vi "בדיקת מתח שחרור של סליל פיקוד ללא עומס 4.vi"(7 "resultUserPrompt":bool=TRUE, 8 "error":errorcluster, 11 "Path for Log":path) -> (0 "error out":errorcluster, 1 "מצב ממסר פתוח/סגור":bool, 2 "מתח פתיחת הממסר":dbl format="%.4f", 3 "מתח מוצא מהספק":dbl format="%.4f")   [LabVIEW 2014]
uses:
  <vilib>/DAQmx/create/channels.llb/DAQmx Create Channel (DO-Digital Output).vi
  <vilib>/DAQmx/write.llb/DAQmx Write (Digital Bool 1Line 1Point).vi
panel:
  out "progress":dbl(slide) scale=0.0..11.0
  out "error IO DMM":errorcluster
  in  "Stop Button":bool
  # "Right-Click to\nexplain error"
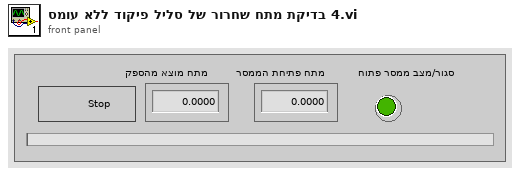
[diagram p1: front panel]
types:
  T1 = enum32{"Invalid", "Standard", "Closed", "Hidden", "Minimized", "Maximized"}
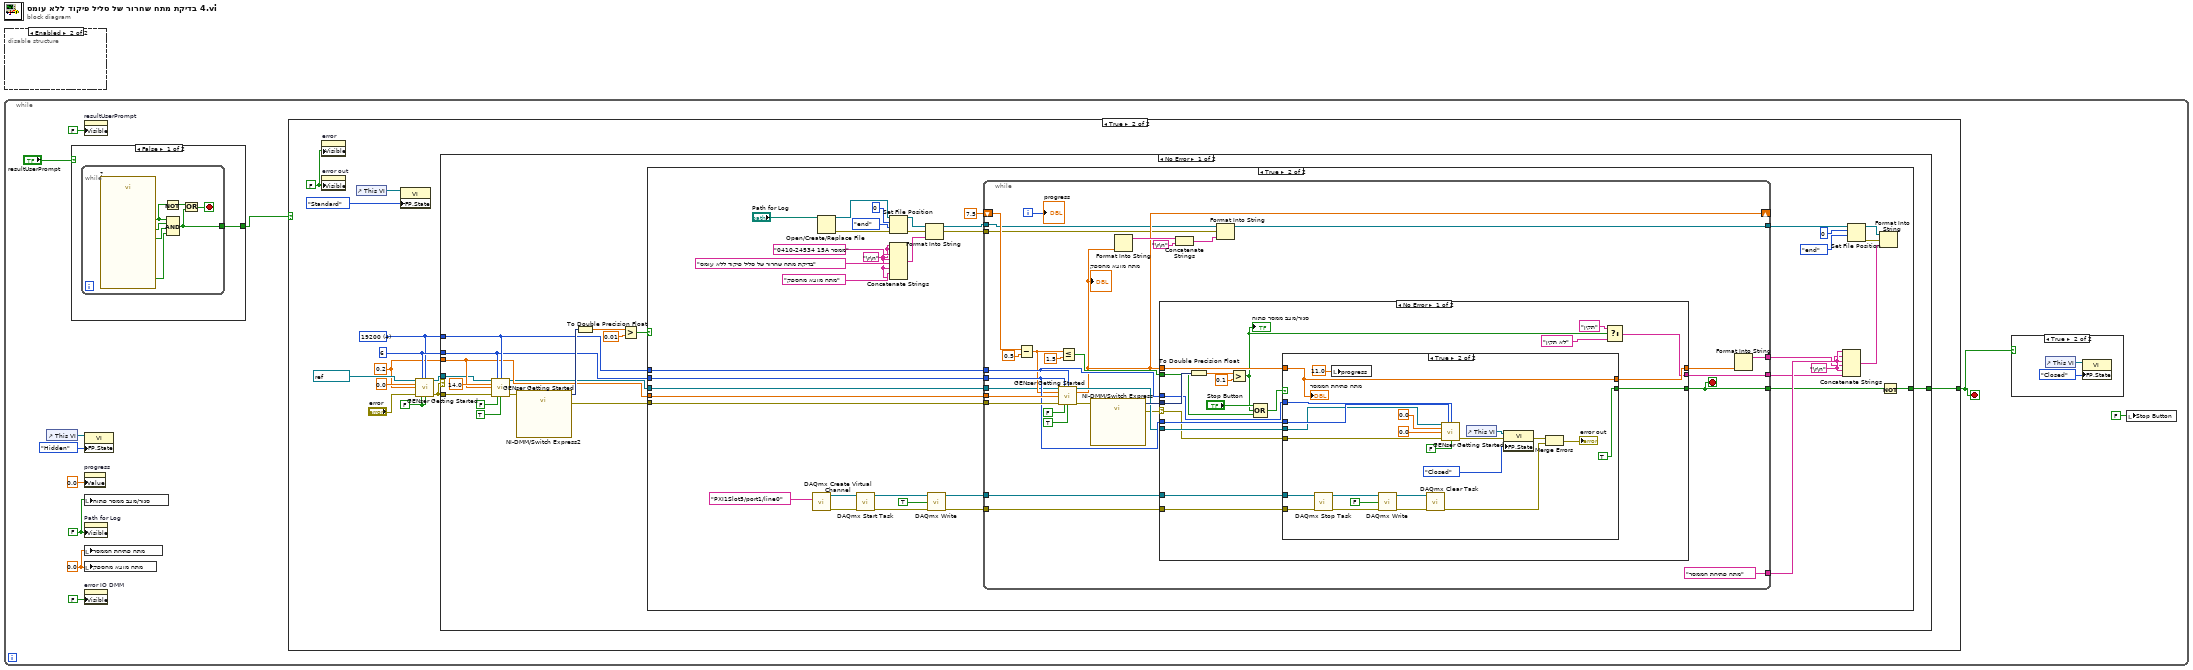
[diagram p0: block diagram]
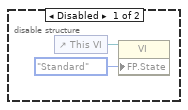
[diagram p2: hidden frame]
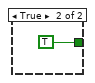
[diagram p4: hidden frame]
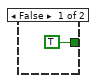
[diagram p5: hidden frame]
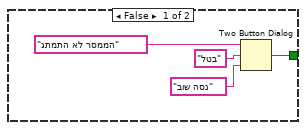
[diagram p6: hidden frame]
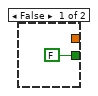
[diagram p7: hidden frame]
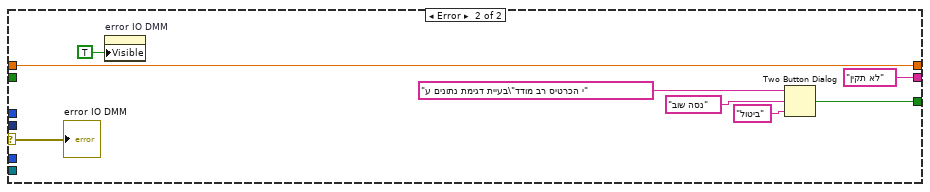
[diagram p8: hidden frame]
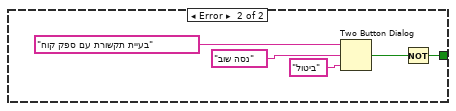
[diagram p9: hidden frame]
diagram:
  n1 = disable-structure shown="Enabled" {
    frame Disabled {
      n2 = control-ref of="This VI"() -> (w1:refnum<vi>)
      n3 = property class="VI"(reference=w1, "FP.State"=T1."Standard" ("Front Panel Window:State")) -> ()  [unwired: 1 in, 2 out]
    }
    frame Enabled {
    }
  }
  n4 = while {
    stop <- w3 stop-if-true
    w7 = FALSE ("מגע סגור")
    w10 = 0.0 ("signals out")
    n5 = control-ref of="This VI"() -> (w9:refnum<vi>)
    n6 = case shown="False" "resultUserPrompt" {
      tunnel: [w16 TRUE] -> w4
      frame False {
        n7 = while {
          tunnel: [w17] -> w16
          stop <- w20 stop-if-true
          n8 = call "?"() -> ("הדקי הרב מודד"=w21:bool, "(מגע שלילי (מעטפת"=w22:bool, "A מגע חיובי"=w23:bool, "OK"=w18:bool)  [unwired: 15 in, 1 out]
          n9 = Not(x=w18) -> (.not. x?=w19:bool)
          n10 = Compound Arithmetic op=AND(w18, w23, w22, w21) -> (w17:bool)
          n11 = Or(x=w19, y=w17) -> (x .or. y?=w20:bool)
        }
      }
      frame True {
      }
    }
    n12 = property on="resultUserPrompt" class="Bool (strict)"("Visible"=FALSE) -> ()  [unwired: 2 in, 2 out]
    n13 = property class="VI"(reference=w9, "FP.State"=T1."Hidden" ("Front Panel Window:State")) -> ()  [unwired: 1 in, 2 out]
    n14 = property on="progress" class="Slide (strict)"("Value"=0.0 ("progress")) -> ()  [unwired: 2 in, 2 out]
    n15 = local write "מצב ממסר פתוח/סגור"(w7) -> ()
    n16 = property on="Path for Log" class="Path"("Visible"=w7) -> ()  [unwired: 2 in, 2 out]
    n17 = local write "מתח פתיחת הממסר"(w10) -> ()
    n18 = local write "מתח מוצא מהספק"(w10) -> ()
    n19 = property on="error IO DMM" class="Clust (strict)"("Visible"=FALSE) -> ()  [unwired: 2 in, 2 out]
    n20 = case shown="True" w4 {
      tunnel: [TRUE ("T button?") w30] -> w3
      frame False {
      }
      frame True {
        w28 = FALSE ("Visible")
        w29 = FALSE ("Output On (T)")
        w34 = u16 4 items=["1200", "2400", "4800", "9600", "19200"] ("BAUD")
        w35 = i16 6 ("GEN Addr")
        w31 = 0.2 ("Current Limit")
        n21 = property on="error" class="Clust (strict)"("Visible"=w28) -> ()  [unwired: 2 in, 2 out]
        n22 = property on="error out" class="Clust (strict)"("Visible"=w28) -> ()  [unwired: 2 in, 2 out]
        n23 = control-ref of="This VI"() -> (w26:refnum<vi>)
        n24 = property class="VI"(reference=w26, "FP.State"=T1."Standard" ("Front Panel Window:State")) -> ()  [unwired: 1 in, 2 out]
        n25 = call "GENser Getting Started.vi"("VISA"=refnum<visa-resource-name> "COM6", "GEN Addr"=w35, "BAUD"=w34, "Voltage Limit"=0.0, "Current Limit"=w31, "error"="error", "Reset (T)"=w29, "Output On (T)"=w29) -> ("VISA out"=w36:refnum<visa-resource-name>, "error out"=w37:errorcluster)  [unwired: 4 in, 2 out]
        n26 = case shown="No Error" w37 {
          tunnel: w37 -> [w47 _]
          tunnel: w36 -> [w43 _]
          tunnel: w35 -> [w45 _]
          tunnel: w34 -> [w46 _]
          tunnel: w31 -> [w44 _]
          tunnel: [w39 w182] -> w30
          frame No Error {
            n27 = call "GENser Getting Started.vi"("VISA"=w43, "GEN Addr"=w45, "BAUD"=w46, "Voltage Limit"=14.0, "Current Limit"=w44, "error"=w47, "Reset (T)"=FALSE, "Output On (T)"=TRUE) -> ("VISA out"=w42:refnum<visa-resource-name>, "error out"=w51:errorcluster)  [unwired: 4 in, 2 out]
            n28 = call "NI-DMM/Switch Express2"("error in"=w51) -> ("signals out"=w50:dynamicdata, "error out"=w48:errorcluster)  [unwired: 16 in, 1 out]
            n29 = To Double Precision Float(number=w50) -> (double precision float=w41:dbl)
            n30 = Greater?(x=w41, y=0.01) -> (0:w49:bool)
            n31 = case shown="True" w49 {
              tunnel: w48 -> [_ w98]
              tunnel: w45 -> [_ w97]
              tunnel: w46 -> [_ w96]
              tunnel: w44 -> [_ w95]
              tunnel: w42 -> [_ w93]
              tunnel: [w55 w59] -> w39
              frame False {
                n32 = Two Button Dialog(message="הממסר לא התמתג", 1:"נסה שוב" ("T button name (\"OK\")"), 2:"בטל" ("T button name (\"OK\")")) -> (T button?=w55:bool)
              }
              frame True {
                w69 = "\r\n"
                w92 = "\r\n"
                n33 = call-poly <vilib>:"DAQmx Create Virtual Channel.vi"("lines"=tag "PXI1Slot5/port1/line0") -> ("task out"=w67:refnum<k21>, "error out"=w68:errorcluster)  [unwired: 13 in]
                n34 = Open/Create/Replace File(file path (use dialog)="Path for Log") -> (refnum out=w80:refnum<file>, error out=w79:errorcluster)  [unwired: 5 in, 1 out]
                n35 = call <vilib>:"DAQmx Start Task.vi"("task/channels in"=w67, "error in"=w68) -> ("task out"=w65:refnum<k21>, "error out"=w64:errorcluster)  [unwired: 12 in]
                n36 = Set File Position(offset (in bytes) (0)=i64 0, refnum=w80, from (0:start)=enum16{"start", "end", "current"}."end", error in=w79) -> (refnum out=w75:refnum<file>, error out=w70:errorcluster)
                n37 = Concatenate Strings(w69, w69, "0410-24534 15A ממסר", w69, "בדיקת מתח שחרור של סליל פיקוד ללא עומס", w69, "מתח מוצא מהספק", w69) -> (w78:string)
                n38 = Format Into String(initial string=w75, error in=w70, w78) -> (resulting string=w72:refnum<file>, error out=w71:errorcluster)  [unwired: 1 in]
                n39 = call-poly <vilib>:"DAQmx Write.vi"("task/channels in"=w65, "data"=TRUE, "error in"=w64) -> ("task out"=w62:refnum<k21>, "error out"=w61:errorcluster)  [unwired: 10 in, 1 out]
                n40 = while {
                  tunnel: w98 -> [w129]
                  tunnel: w97 -> [w122]
                  tunnel: w96 -> [w121]
                  tunnel: w95 -> [w127]
                  shift-right: [w104] -> _
                  shift-left: 7.5 ("y") -> [w125]
                  tunnel: w93 -> [w114]
                  tunnel: [w109] -> w87
                  tunnel: ["מתח פתיחת הממסר"] -> w86
                  tunnel: [w107] -> w85
                  tunnel: [w106] -> w84
                  tunnel: w72 -> [w103]
                  tunnel: w71 -> [w102]
                  tunnel: w62 -> [w101]
                  tunnel: w61 -> [w100]
                  tunnel: [w99] -> w60
                  i -> [w115]
                  stop <- w99 stop-if-true
                  n41 = Subtract(x=w125, y=0.5) -> (x-y=w118:dbl)
                  n42 = call "GENser Getting Started.vi"("VISA"=w114, "GEN Addr"=w122, "BAUD"=w121, "Voltage Limit"=w118, "Current Limit"=w127, "error"=w129, "Reset (T)"=FALSE, "Output On (T)"=TRUE) -> ("VISA out"=w120:refnum<visa-resource-name>, "Output Voltage"=w104:dbl, "error out"=w124:errorcluster)  [unwired: 4 in, 1 out]
                  "מתח מוצא מהספק" <- w104
                  n43 = Less Or Equal?(x=w118, y=1.5) -> (x <= y?=w117:bool)
                  n44 = call "NI-DMM/Switch Express"("error in"=w124) -> ("signals out"=w123:dynamicdata, "error out"=w116:errorcluster)  [unwired: 16 in, 1 out]
                  n45 = Format Into String(w104) -> (resulting string=w111:string)  [unwired: 3 in, 1 out]
                  n46 = case shown="No Error" w116 {
                    selector: w116 -> [w139 w180]
                    tunnel: w123 -> [w148 _]
                    tunnel: [w145 w176] -> w99
                    tunnel: w122 -> [w144 _]
                    tunnel: w121 -> [w143 _]
                    tunnel: w120 -> [w142 _]
                    tunnel: w117 -> [w141 _]
                    tunnel: w104 -> [w140 w174]
                    tunnel: [w133 w174] -> w110
                    tunnel: [w132 "לא תקין"] -> w106
                    tunnel: w101 -> [w131 _]
                    tunnel: w100 -> [w130 _]
                    frame No Error {
                      n47 = To Double Precision Float(number=w148) -> (double precision float=w138:dbl)
                      n48 = Greater?(x=w138, y=0.1) -> (0:w134:bool)
                      "מצב ממסר פתוח/סגור" <- w134
                      n49 = Compound Arithmetic op=OR("Stop Button", w134, w141) -> (w147:bool)
                      n50 = case shown="True" w147 {
                        tunnel: [FALSE TRUE] -> w145
                        tunnel: w144 -> [_ w171]
                        tunnel: w143 -> [_ w170]
                        tunnel: w142 -> [_ w169]
                        tunnel: w139 -> [_ w166]
                        tunnel: w140 -> [_ w160]
                        tunnel: [_ w160] -> w133
                        tunnel: w131 -> [_ w154]
                        tunnel: w130 -> [_ w153]
                        frame False {
                        }
                        frame True {
                          n51 = call <vilib>:"DAQmx Stop Task.vi"("task/channels in"=w154, "error in"=w153) -> ("task out"=w159:refnum<k21>, "error out"=w158:errorcluster)  [unwired: 12 in]
                          n52 = local write "progress"(11.0 ("progress")) -> ()
                          n53 = call-poly <vilib>:"DAQmx Write.vi"("task/channels in"=w159, "data"=FALSE, "error in"=w158) -> ("task out"=w157:refnum<k21>, "error out"=w156:errorcluster)  [unwired: 10 in, 1 out]
                          n54 = call <vilib>:"DAQmx Clear Task.vi"("task in"=w157, "error in"=w156) -> ("error out"=w152:errorcluster)  [unwired: 13 in]
                          n55 = call "GENser Getting Started.vi"("VISA"=w169, "GEN Addr"=w171, "BAUD"=w170, "Voltage Limit"=0.0, "Current Limit"=0.0, "error"=w166, "Output On (T)"=FALSE) -> ("error out"=w161:errorcluster)  [unwired: 5 in, 3 out]
                          n56 = control-ref of="This VI"() -> (w162:refnum<vi>)
                          n57 = property class="VI"(reference=w162, error in=w161, "FP.State"=T1."Closed" ("Front Panel Window:State")) -> (error out=w151:errorcluster)  [unwired: 1 out]
                          n58 = Merge Errors(w151, w152) -> (→"error out":errorcluster)
                          "מתח פתיחת הממסר" <- w160
                        }
                      }
                      n59 = Select(t="תקין", s=w134, f="לא תקין") -> (s? t:f=w132:string)
                    }
                    frame Error {
                      n60 = property on="error IO DMM" class="Clust (strict)"("Visible"=TRUE) -> ()  [unwired: 2 in, 2 out]
                      n61 = Two Button Dialog(message="בעיית דגימת נתונים ע\"י הכרטיס רב מודד", 1:"ביטול" ("F button name (\"Cancel\")"), 2:"נסה שוב" ("T button name (\"OK\")")) -> (T button?=w176:bool)
                      "error IO DMM" <- w180
                    }
                  }
                  n62 = Concatenate Strings(w111, "\r\n") -> (w105:string)
                  n63 = Format Into String(initial string=w103, error in=w102, w105) -> (resulting string=w109:refnum<file>)  [unwired: 1 in, 1 out]
                  n64 = Format Into String(w110) -> (resulting string=w107:string)  [unwired: 3 in, 1 out]
                  "progress" <- w115
                }
                n65 = Concatenate Strings(w92, w86, w92, w85, w92, w84) -> (w83:string)
                n66 = Set File Position(offset (in bytes) (0)=i64 0, refnum=w87, from (0:start)=enum16{"start", "end", "current"}."end") -> (refnum out=w89:refnum<file>, error out=w88:errorcluster)  [unwired: 1 in]
                n67 = Format Into String(initial string=w89, error in=w88, w83) -> ()  [unwired: 1 in, 2 out]
                n68 = Not(x=w60) -> (.not. x?=w59:bool)
              }
            }
          }
          frame Error {
            n69 = Two Button Dialog(message="בעיית תקשורת עם ספק קוח", 1:"ביטול" ("F button name (\"Cancel\")"), 2:"נסה שוב" ("T button name (\"OK\")")) -> (T button?=w181:bool)
            n70 = Not(x=w181) -> (.not. x?=w182:bool)
          }
        }
      }
    }
    n71 = case shown="True" w3 {
      frame False {
      }
      frame True {
        n72 = control-ref of="This VI"() -> (w15:refnum<vi>)
        n73 = property class="VI"(reference=w15, "FP.State"=T1."Closed" ("Front Panel Window:State")) -> ()  [unwired: 1 in, 2 out]
      }
    }
    n74 = local write "Stop Button"(FALSE ("Reset (T)")) -> ()
  }
